vi "invoke reentrant method in parallel.vi"(4 "results reporter":refnum<class "results reporter.lvclass">, 5 "execution system":T1=enum."standard", 6 "task token":refnum<class "null task token.lvclass">, 7 "IDs":string[](array[string]), 8 "error in":errorcluster, 9 "parameters":variant[](array[variant]), 10 "VI in":T2, 11 "dispatcher":refnum<data-value>) -> (0 "error out":errorcluster, 3 "dispatcher out":refnum<data-value>)   [LabVIEW 2013, in "call by reference action.lvclass"]
uses:
  call by reference action.lvclass
  function definition.ctl
  task token/null task token.lvclass
  dispatcher/thread pool.lvclass
  dispatcher/execution system.ctl
  results reporter/results reporter.lvclass
  standard tasks/batch task/reporting type.ctl
  standard tasks/batch task/batch task.lvclass
  close reference reporter/close reference and report.lvclass
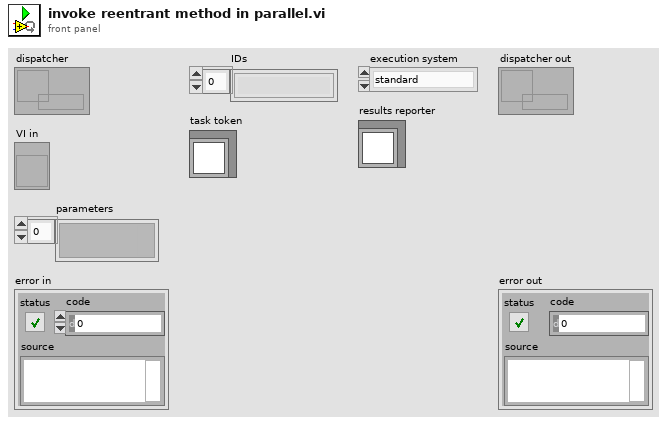
[diagram p1: front panel]
types:
  T1 = typedef "thread pool.lvclass/execution system.ctl" = enum32{"user interface", "standard", "instrument i/o", "data acquisition", "other 1", "other 2"}
  T2 = typedef "call by reference action.lvclass/function definition.ctl" = refnum<vi>
  T3 = typedef "batch task.lvclass/reporting type.ctl" = enum16{"return immediately", "wait on all"}
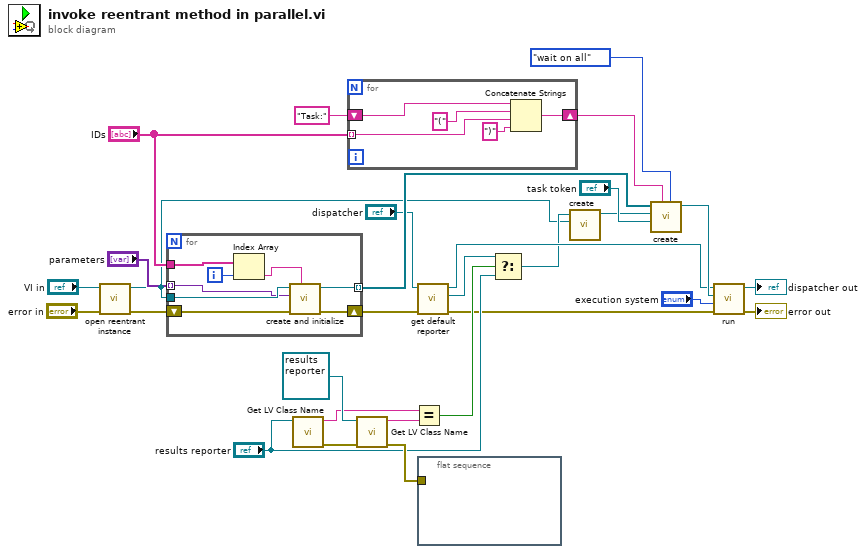
[diagram p0: block diagram]
diagram:
  n1 = call "open reentrant instance.vi"("error in"="error in", "function"="VI in") -> ("error out"=w23:errorcluster, "reentrant instance"=w1:T2)  [unwired: 8 in]
  n2 = for {
    tunnel: w1 -> [w35]
    shift-right: [w37] -> w9
    shift-left: w23 -> [w36]
    tunnel: "parameters" -> [w34] mode=indexing
    tunnel: [w33] -> w21 mode=indexing
    tunnel: "IDs" -> [w30]
    i -> [w32]
    n3 = Index Array(array=w30, index=w32) -> (element=w31:string)
    n4 = call "create and initialize.vi"("action name"=w31, "error in"=w36, "parameters"=w34, "function"=w35) -> ("error out"=w37:errorcluster, "call by reference action"=w33:refnum<class "call by reference action.lvclass">)  [unwired: 6 in]
  }
  n5 = call <vilib>:"Get LV Class Name.vi"("object"="results reporter") -> ("error out"=w15:errorcluster, "class name"=w13:string)  [unwired: 9 in]
  n6 = for {
    tunnel: "IDs" -> [w42] mode=indexing
    shift-right: [w39] -> w18
    shift-left: "Task:" -> [w38]
    n7 = Concatenate Strings(w38, "(" ("string"), w42, ")" ("string")) -> (w39:string)
  }
  n8 = call <vilib>:"Get LV Class Name.vi"("error in (no error)"=w15, "object"=refnum<class "results reporter.lvclass"> refnum ("results reporter")) -> ("error out"=w12:errorcluster, "class name"=w14:string)  [unwired: 8 in]
  n9 = Equal?(x=w13, y=w14) -> (x = y?=w11:bool)
  n10 = call "get default reporter.vi"("error in"=w9, "dispatcher"="dispatcher") -> ("error out"=w8:errorcluster, "default result reporter"=w5:refnum<class "results reporter.lvclass">, "dispatcher out"=w6:refnum<data-value>)  [unwired: 7 in]
  n11 = flat-sequence {
    tunnel: w12 -> [_]
    frame #0 {
    }
  }
  n12 = Select(t=w5, s=w11, f="results reporter") -> (s? t:f=w3:refnum<class "results reporter.lvclass">)
  n13 = call "create.vi"("reference to close"=w1, "original reporter"=w3) -> ("close reference and report out"=w4:refnum<class "close reference and report.lvclass">)  [unwired: 9 in]
  n14 = call "create.vi"("reporting type"=reporting_type."wait on all", "ID"=w18, "task token"="task token", "results reporter"=w4, "actions"=w21) -> ("batch task out"=w27:refnum<class "batch task.lvclass">)  [unwired: 6 in]
  n15 = call "run.vi"("error in"=w8, "execution system"="execution system", "task"=w27, "dispatcher"=w6) -> ("error out"=→"error out":errorcluster, "dispatcher out"=→"dispatcher out":refnum<data-value>)  [unwired: 6 in]
